vi "Destroy.vi"(0 "reference in":refnum<class "Master Controller.lvclass">, 5 "error in (no error)":errorcluster) -> (14 "reference out":refnum<class "Master Controller.lvclass">, 19 "error out":errorcluster)   [LabVIEW 2015, in "Master Controller.lvclass"]
doc: "Destructor."
uses:
  Master Controller.lvclass
  GUI/GUI Controller_llb/GUI Controller.lvclass
  File Controller_llb/File Controller.lvclass
  Subject Controller_llb/Subject Controller.lvclass
  <vilib>/addons/_AddQ/G#Object/G#Object.lvclass
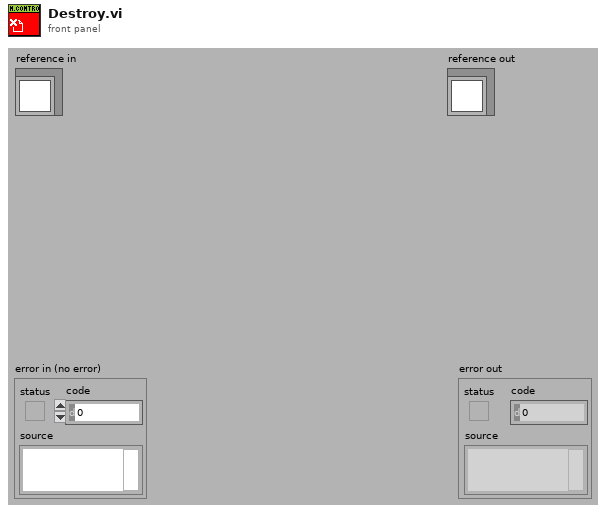
[diagram p1: front panel]
types:
  T1 = typedef "Master Controller.lvclass/ObjectAttributes.ctl" = cluster{"MyAttribute":dbl, "gui_controller_ref":refnum<class "GUI Controller.lvclass">, "file_controller_ref":refnum<class "File Controller.lvclass">, "subject_controller_ref":refnum<class "Subject Controller.lvclass">}
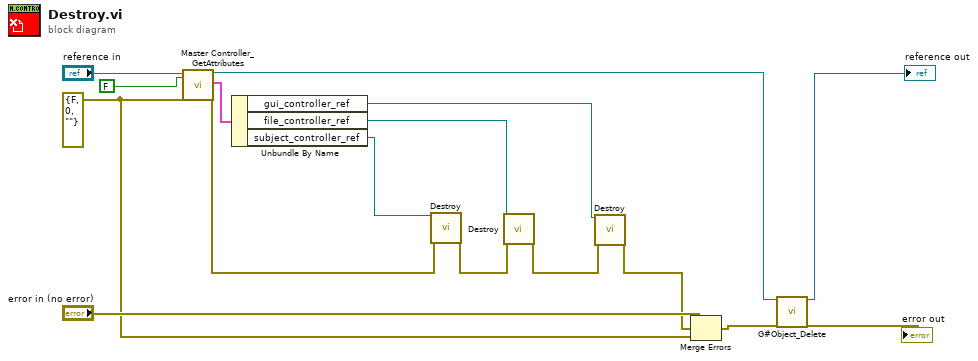
[diagram p0: block diagram]
diagram:
  w14 = errorcluster {"status"=FALSE, "code"=0, "source"=""} ("error in (no error)")
  n1 = call "Master Controller_GetAttributes.vi"("reference in"="reference in", "return data? (T)"=FALSE ("simple info"), "error in (no error)"=w14) -> ("reference out"=w11:refnum<class "Master Controller.lvclass">, "attributes"=w8:T1, "error out"=w4:errorcluster)  [unwired: 13 in, 1 out]
  n2 = Unbundle By Name(w8) -> ("gui_controller_ref"=w7:refnum<class "GUI Controller.lvclass">, "file_controller_ref"=w6:refnum<class "File Controller.lvclass">, "subject_controller_ref"=w5:refnum<class "Subject Controller.lvclass">)
  n3 = call-dynamic "Destroy.vi"("reference in"=w5, "error in (no error)"=w4) -> ("error out"=w3:errorcluster)  [unwired: 16 in, 1 out]
  n4 = call-dynamic "Destroy.vi"("reference in"=w6, "error in (no error)"=w3) -> ("error out"=w2:errorcluster)  [unwired: 16 in, 1 out]
  n5 = call-dynamic "Destroy.vi"("reference in"=w7, "error in (no error)"=w2) -> ("error out"=w1:errorcluster)  [unwired: 16 in, 1 out]
  n6 = Merge Errors("error in (no error)", w1, w14) -> (w13:errorcluster)
  n7 = call <vilib>:"G#Object_Delete.vi"("reference in"=w11, "error in (no error)"=w13) -> ("reference out"=→"reference out":refnum<class "Master Controller.lvclass">, "error out"=→"error out":errorcluster)  [unwired: 16 in]
